vi "VNARP-BOXCAR.vi"(3 "Y IN":dbl[](array[numeric]), 4 "kernel size (pts)":i32=25, 5 "Freq table IN":dbl[](array[numeric])) -> (0 "Y OUT":dbl[](array[numeric]), 2 "Freq table OUT":dbl[](array[numeric]))   [LabVIEW 2021]
uses:
  <vilib>/Analysis/2dsp.llb/1D Convolution (DBL).vi
  <vilib>/Analysis/NI_AALPro.lvlib
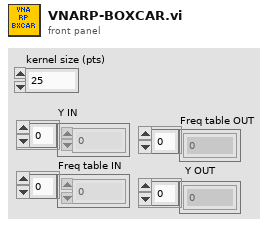
[diagram p1: front panel]
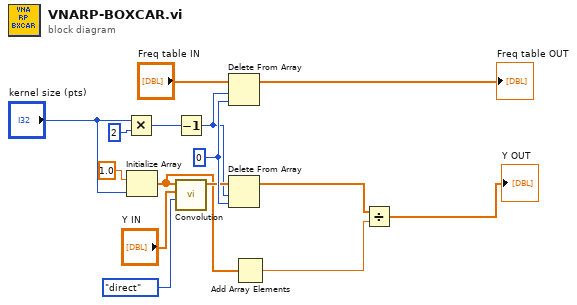
[diagram p0: block diagram]
diagram:
  w14 = 0 ("indice")
  n1 = Multiply(x="kernel size (pts)", y=2) -> (x*y=w11:i32)
  n2 = Initialize Array(1.0 ("élément"), "kernel size (pts)") -> (w4:dbl[])
  n3 = Decrement(x=w11) -> (x-1=w7:i32)
  n4 = call-poly <vilib>:"Convolution.vi"("algorithm"=enum32{"direct", "frequency domain"}."direct", "Y"="Y IN", "X"=w4) -> ("X * Y"=w12:dbl[])  [unwired: 7 in, 1 out]
  n5 = Delete From Array(array="Freq table IN", length=w7, index=w14) -> (array with subset deleted=→"Freq table OUT":dbl[])  [unwired: 1 out]
  n6 = Delete From Array(array=w12, length=w7, index=w14) -> (array with subset deleted=w2:dbl[])  [unwired: 1 out]
  n7 = Add Array Elements(numeric array=w4) -> (sum=w3:dbl)
  n8 = Divide(x=w2, y=w3) -> (x/y=→"Y OUT":dbl[])
